vi "Set Clip Plane (reference).vi"(8 "error in (no error)":errorcluster, 9 "Clip Plane State":enum16{"Inherit Value", "Off", "On"}(ring), 10 "Clip Plane Refnum In":refnum<vi>, 11 "Scene Object In":refnum<vi>) -> (0 "error out":errorcluster, 2 "Clip Plane Refnum Out":refnum<vi>, 3 "Scene Object Out":refnum<vi>)   [LabVIEW 2020, in "NI_3D Picture Control.lvlib"]
doc: "Defines the plane beyond which LabVIEW clips, or does not render, surfaces in a scene."
uses:
  <vilib>/picture/3D Picture Control/NI_3D Picture Control.lvlib
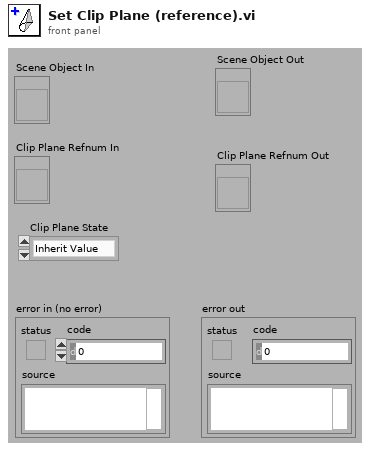
[diagram p1: front panel]
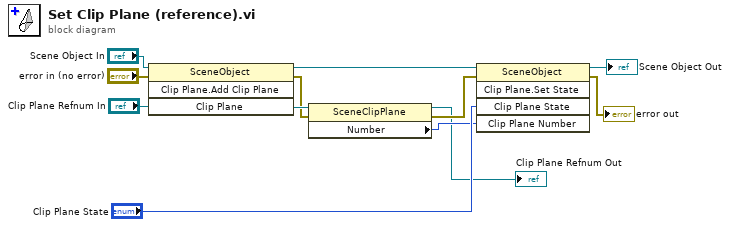
[diagram p0: block diagram]
diagram:
  n1 = invoke class="SceneObject" method="Clip Plane.Add Clip Plane"(reference="Scene Object In", error in="error in (no error)", "Clip Plane"="Clip Plane Refnum In") -> (reference out=w8:refnum<vi>, error out=w3:errorcluster, "Clip Plane"=w5:refnum<vi>)  [unwired: 1 in, 1 out]
  n2 = property class="SceneClipPlane"(reference=w5, error in=w3) -> (reference out=→"Clip Plane Refnum Out":refnum<vi>, error out=w2:errorcluster, "Number"=w4:i32)
  n3 = invoke class="SceneObject" method="Clip Plane.Set State"(reference=w8, error in=w2, "Clip Plane State"="Clip Plane State", "Clip Plane Number"=w4) -> (reference out=→"Scene Object Out":refnum<vi>, error out=→"error out":errorcluster)  [unwired: 1 in, 3 out]
